vi "send_to_dds.vi"(7 "inversion selector":T2(ring), 11 "synthesizer point":T1) -> ()   [LabVIEW 2010]
uses:
  synthesizer_point_cluster.ctl
  <vilib>/eio/EIONode/EIONode.xnode
  <vilib>/rvi/eio/nirviEIOImplementation/nirviEIOImplementation.xnode
  <vilib>/rvi/eio/common/nirviEmuClasses.ctl
  <vilib>/rvi/eio/common/nirviEmuTemplateMethod_noerrors.vi
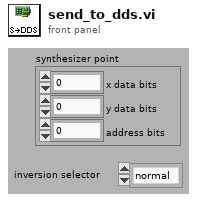
[diagram p1: front panel]
types:
  T1 = typedef "synthesizer_point_cluster.ctl" = cluster{"x data bits":u8, "y data bits":u8, "address bits":u8}
  T2 = enum16{"normal", "x inversed", "y inversed", "x & y inversed"}
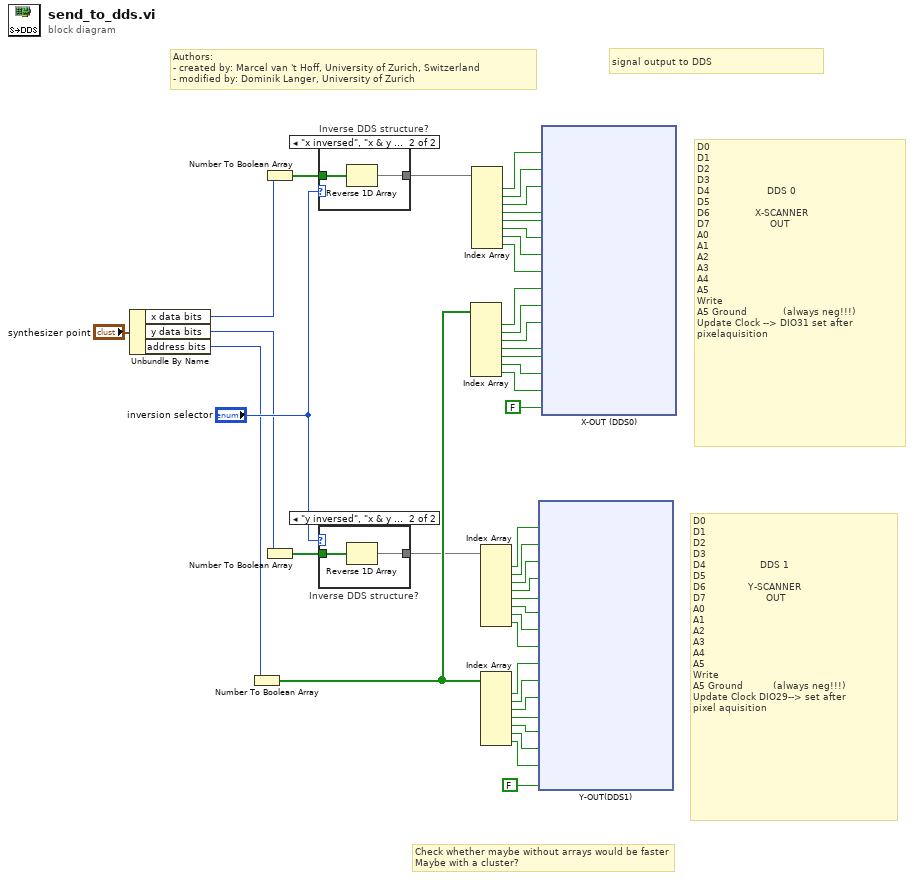
[diagram p0: block diagram]
diagram:
  # "Check whether maybe without arrays would be faster\nMaybe with a cluster?"
  # "D0                                     \nD1\nD2\nD3                        \nD4                  DDS 1\nD5\nD6              Y-SCANNER\nD7                    OUT\nA0\nA1\nA2\nA3\nA4\nA5\nWrite  \nA5 Ground          (always neg!!!)\nUpdate Clock DIO29--> set after \npixel aquisition"
  # "D0                                      \nD1\nD2\nD3                        \nD4                   DDS 0\nD5                  \nD6               X-SCANNER\nD7                    OUT\nA0\nA1\nA2\nA3\nA4\nA5\nWrite\nA5 Ground            (always neg!!!) \nUpdate Clock --> DIO31 set after \npixelaquisition"
  # "Authors: \n- created by: Marcel van 't Hoff, University of Zurich, Switzerland\n- modified by: Dominik Langer, University of Zurich"
  # "signal output to DDS"
  n1 = Unbundle By Name("synthesizer point") -> ("x data bits"=w3:u8, "y data bits"=w2:u8, "address bits"=w1:u8)
  n2 = Number To Boolean Array(number=w1) -> (Boolean array=w17:bool[])
  n3 = Number To Boolean Array(number=w3) -> (Boolean array=w6:bool[])
  n4 = Number To Boolean Array(number=w2) -> (Boolean array=w9:bool[])
  n5 = case "Inverse DDS structure?" shown="\"x inversed\", \"x & y inversed\"" "inversion selector" {
    tunnel: [w43 w44] -> w5
    tunnel: w6 -> [w43 w45]
    frame Default {
    }
    frame "x inversed", "x & y inversed" {
      n6 = Reverse 1D Array(array=w45) -> (reversed array=w44:bool[])
    }
  }
  n7 = case "Inverse DDS structure?" shown="\"y inversed\", \"x & y inversed\"" "inversion selector" {
    tunnel: [w46 w47] -> w8
    tunnel: w9 -> [w46 w48]
    frame Default {
    }
    frame "y inversed", "x & y inversed" {
      n8 = Reverse 1D Array(array=w48) -> (reversed array=w47:bool[])
    }
  }
  n9 = Index Array(array=w17) -> (element #1=w40:bool, element #2=w39:bool, element #3=w38:bool, element #4=w37:bool, element #5=w36:bool, element #6=w35:bool, element #7=w34:bool)  [unwired: 7 in]
  n10 = Index Array(array=w5) -> (element #1=w33:bool, element #2=w32:bool, element #3=w31:bool, element #4=w30:bool, element #5=w29:bool, element #6=w28:bool, element #7=w27:bool, element #8=w26:bool)  [unwired: 8 in]
  n11 = Index Array(array=w8) -> (element #1=w25:bool, element #2=w24:bool, element #3=w23:bool, element #4=w22:bool, element #5=w21:bool, element #6=w20:bool, element #7=w19:bool, element #8=w18:bool)  [unwired: 8 in]
  n12 = Index Array(array=w17) -> (element #1=w16:bool, element #2=w15:bool, element #3=w14:bool, element #4=w13:bool, element #5=w12:bool, element #6=w11:bool, element #7=w10:bool)  [unwired: 7 in]
  n13 = xnode "Y-OUT(DDS1)"("Connector3/DIO0"=w25, "Connector3/DIO1"=w24, "Connector3/DIO2"=w23, "Connector3/DIO3"=w22, "Connector3/DIO4"=w21, "Connector3/DIO5"=w20, "Connector3/DIO6"=w19, "Connector3/DIO7"=w18, "Connector3/DIO16"=w16, "Connector3/DIO17"=w15, "Connector3/DIO18"=w14, "Connector3/DIO19"=w13, "Connector3/DIO20"=w12, "Connector3/DIO37"=w11, "Connector3/DIO26"=w10, "Connector3/DIO36"=FALSE) -> ()  [unwired: 16 in, 16 out]
  n14 = xnode "X-OUT (DDS0)"("Connector3/DIO15"=w33, "Connector3/DIO14"=w32, "Connector3/DIO13"=w31, "Connector3/DIO12"=w30, "Connector3/DIO11"=w29, "Connector3/DIO10"=w28, "Connector3/DIO9"=w27, "Connector3/DIO8"=w26, "Connector3/DIO21"=w40, "Connector3/DIO22"=w39, "Connector3/DIO23"=w38, "Connector3/DIO24"=w37, "Connector3/DIO25"=w36, "Connector3/DIO35"=w35, "Connector3/DIO27"=w34, "Connector3/DIO34"=FALSE) -> ()  [unwired: 16 in, 16 out]
